vi "Global_init.vi"(11 "error in":errorcluster) -> (3 "error out":errorcluster)   [LabVIEW 2026]
uses:
  GlobalVariable/Muestreo.vi
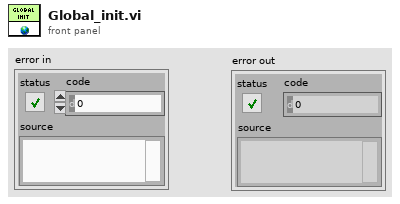
[diagram p1: front panel]
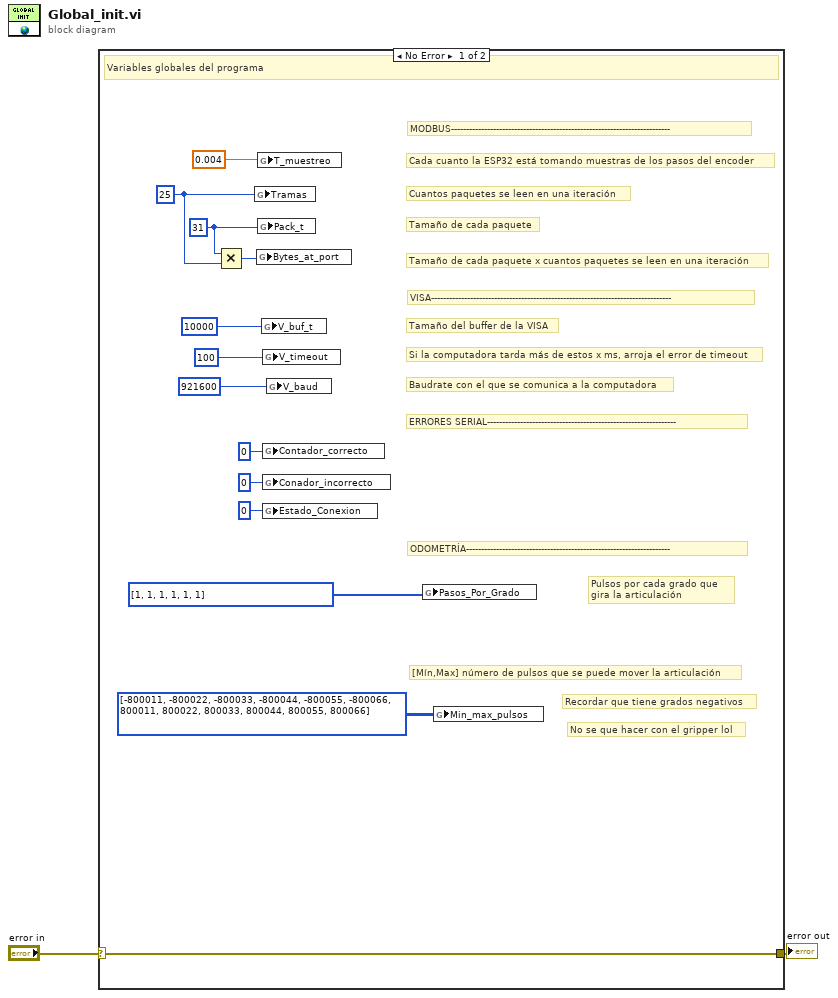
[diagram p0: block diagram]
diagram:
  n1 = case shown="No Error" "error in" {
    selector: "error in" -> [w12 w16]
    tunnel: [w12 w16] -> w1
    frame No Error {
      w9 = 25 ("Tramas")
      w13 = 31 ("Pack_t")
      # "No se que hacer con el gripper lol"
      # "Recordar que tiene grados negativos"
      # "[Mín,Max] número de pulsos que se puede mover la articulación"
      # "Pulsos por cada grado que gira la articulación"
      # "ODOMETRÍA--------------------------------------------------------------------"
      # "ERRORES SERIAL---------------------------------------------------------------"
      # "MODBUS-------------------------------------------------------------------------"
      # "Cada cuanto la ESP32 está tomando muestras de los pasos del encoder"
      # "Tamaño de cada paquete x cuantos paquetes se leen en una iteración"
      # "Tamaño de cada paquete"
      # "Cuantos paquetes se leen en una iteración"
      # "Tamaño del buffer de la VISA"
      # "Si la computadora tarda más de estos x ms, arroja el error de timeout"
      # "Baudrate con el que se comunica a la computadora"
      # "VISA--------------------------------------------------------------------------------"
      # "Variables globales del programa"
      n2 = Multiply(x=w13, y=w9) -> (x*y=w14:i32)
      n3 = global write "Muestreo.vi" "Tramas"(w9) -> ()
      n4 = global write "Muestreo.vi" "Bytes_at_port"(w14) -> ()
      n5 = global write "Muestreo.vi" "T_muestreo"(0.004) -> ()
      n6 = global write "Muestreo.vi" "Pack_t"(w13) -> ()
      n7 = global write "Muestreo.vi" "V_buf_t"(u32 10000 ("V_buf_t")) -> ()
      n8 = global write "Muestreo.vi" "V_timeout"(u32 100 ("V_timeout")) -> ()
      n9 = global write "Muestreo.vi" "Contador_correcto"(u32 0 ("V_buf_t")) -> ()
      n10 = global write "Muestreo.vi" "Conador_incorrecto"(u32 0 ("V_timeout")) -> ()
      n11 = global write "Muestreo.vi" "Estado_Conexion"(u32 0 ("V_baud")) -> ()
      n12 = global write "Muestreo.vi" "V_baud"(u32 921600 ("V_baud")) -> ()
      n13 = global write "Muestreo.vi" "Pasos_Por_Grado"(i32[] [1, 1, 1, 1, 1, 1]) -> ()
      n14 = global write "Muestreo.vi" "Min_max_pulsos"(i32[][] [[-800011, -800022, -800033, -800044, -800055, -800066], [800011, 800022, 800033, 800044, 800055, 800066]]) -> ()
    }
    frame Error {
    }
  }
  "error out" <- w1
